vi "DisArmTrigger.vi"(8 "error in":errorcluster, 11 "TriggerBox in":refnum<class "TriggerBox.lvclass">) -> (0 "error out":errorcluster, 3 "TriggerBox out":refnum<class "TriggerBox.lvclass">)   [LabVIEW 2013, in "TriggerBox.lvclass"]
uses:
  TriggerBox.lvclass
  <vilib>/Utility/error.llb/Error Cluster From Error Code.vi
  <vilib>/rvi/errors/niLvFpgaAdjustHostInterfaceError.vi
  RT/FPGASession/FPGARef.ctl
  <vilib>/rvi/interface/nirviReadWriteControl/nirviReadWriteControl.xnode
  FPGA Bitfiles/HWSWTriggerBox_FPGATarget2_TriggerBox_1zhzIx5zPP8.lvbitx
  FPGAMain.vi
  FPGASessionClass/FPGASession.lvclass
  NiFpgaLv.dll
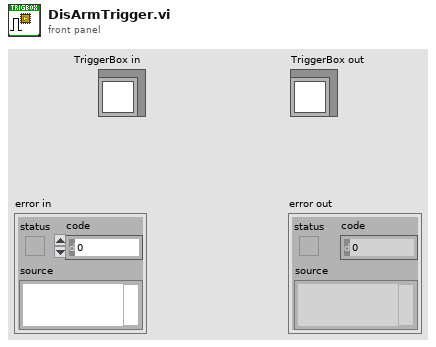
[diagram p1: front panel]
types:
  T1 = typedef "FPGASession.lvclass/FPGARef.ctl" = refnum<k20>
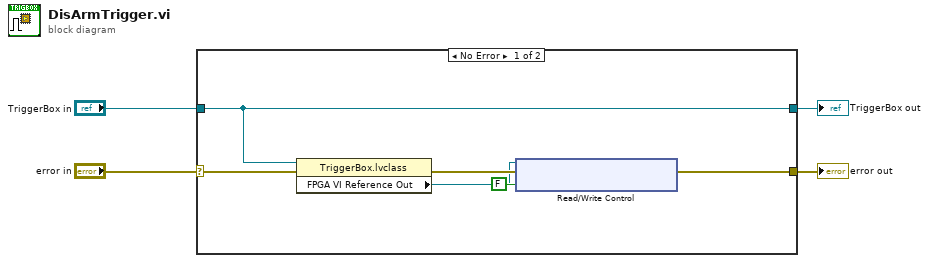
[diagram p0: block diagram]
diagram:
  n1 = case shown="No Error" "error in" {
    selector: "error in" -> [w7 w12]
    tunnel: [w10 w12] -> w1
    tunnel: [w8 w11] -> w2
    tunnel: "TriggerBox in" -> [w8 w11]
    frame No Error {
      n2 = property class="TriggerBox.lvclass"(reference=w8, error in=w7) -> (error out=w6:errorcluster, "FPGA VI Reference Out"=w5:T1)  [unwired: 1 out]
      n3 = xnode "Read/Write Control"("FPGA VI Reference In"=w5, "error in"=w6, "ArmTrigger"=FALSE) -> ("error out"=w10:errorcluster)  [unwired: 1 out]
    }
    frame Error {
    }
  }
  "error out" <- w1
  "TriggerBox out" <- w2
